vi "FTW-Test-JSON-Fuzz.vi"() -> (0 "Test Result":errorcluster)   [LabVIEW 2015]
uses:
  src/error/FTW-ERR-ThrowInfo.vi
  src/error/FTW-ERR-ThrowError.vi
  src/error/FTW-ERR-CallChain.vi
  src/string/FTW-STR-ReplaceWhitespace.vi
  src/string/FTW-STR-Array-Delimit.vi
  src/error/FTW-ERR-Clear.vi
  src/regex/FTW-Regex-ReplaceAll.vi
  codegen/xnode/FTW-Dataflow-Synchronizer.xnode
panel:
  out "JSON String (UTF-8)":string
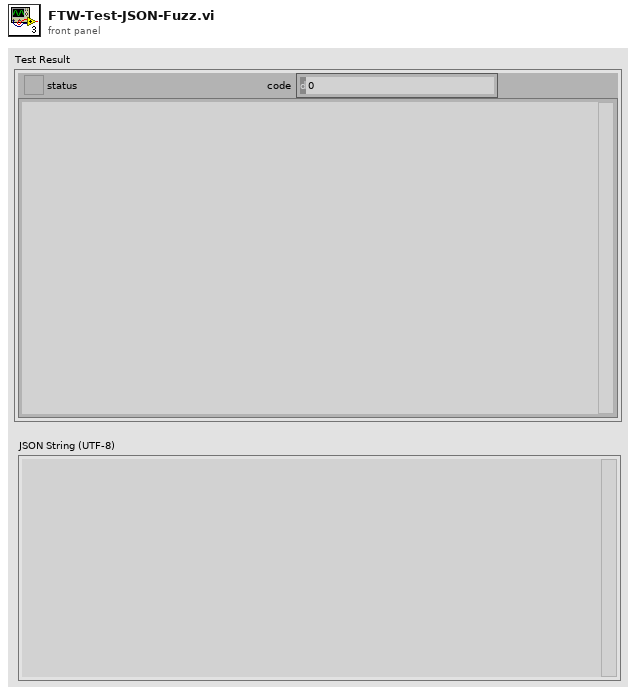
[diagram p1: front panel]
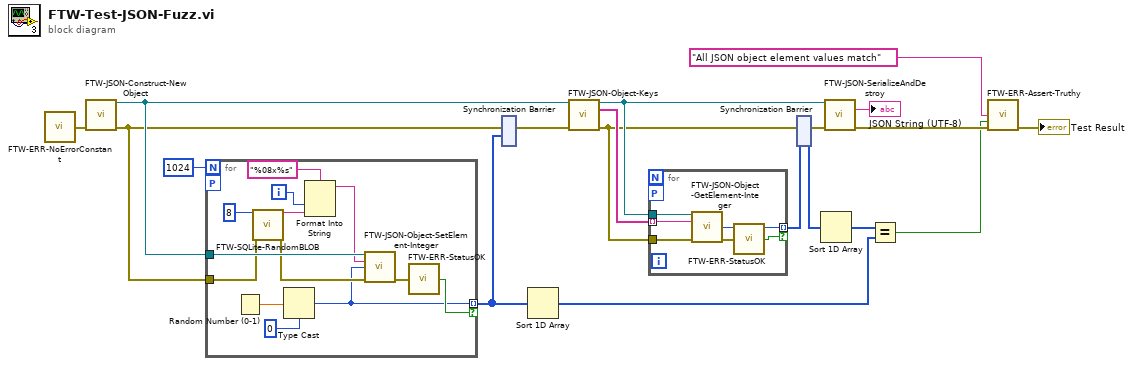
[diagram p0: block diagram]
diagram:
  n1 = call "FTW-ERR-NoErrorConstant.vi"() -> ("no error"=w16:errorcluster)
  n2 = call "FTW-JSON-Construct-NewObject.vi"("error in"=w16) -> ("JSON Object"=w18:refnum<data-value>, "error out"=w9:errorcluster)  [unwired: 13 in]
  n3 = for {
    N: 1024 -> [_]
    workers-P: _ -> [_]
    tunnel: w9 -> [w30]
    tunnel: w18 -> [w32]
    tunnel: [w21] -> w7 mode=indexing if=w23
    i -> [w26]
    n4 = Random Number (0-1)() -> (number: 0 to 1=w22:dbl)
    n5 = call "FTW-SQLite-RandomBLOB.vi"("Number of Bytes"=8, "error in"=w30) -> ("Random BLOB"=w27:string, "error out"=w29:errorcluster)  [unwired: 12 in]
    n6 = Type Cast(type=i64 0, x=w22) -> (*(type *) &x=w21:i64)
    n7 = Format Into String(format string="%08x%s", w26, w27) -> (resulting string=w24:string)  [unwired: 2 in, 1 out]
    n8 = call "FTW-JSON-Object-SetElement-Integer.vi"("JSON Object"=w32, "Key"=w24, "Value"=w21, "error in"=w29) -> ("error out"=w28:errorcluster)  [unwired: 10 in, 1 out]
    n9 = call "FTW-ERR-StatusOK.vi"("error to check"=w28) -> ("Status OK?"=w23:bool)
  }
  n10 = xnode "Synchronization Barrier"("Synchronized Signal 1"=w9, "Synchronized Signal 2"=w7) -> ("error out out"=w8:errorcluster)  [unwired: 1 out]
  n11 = Sort 1D Array(array=w7) -> (sorted array=w13:i64[])
  n12 = call "FTW-JSON-Object-Keys.vi"("JSON Object"=w18, "error in"=w8) -> ("JSON Object out"=w11:refnum<data-value>, "Keys"=w15:string[], "error out"=w6:errorcluster)  [unwired: 11 in]
  n13 = for {
    tunnel: w15 -> [w37] mode=indexing
    tunnel: [w35] -> w4 mode=indexing if=w33
    workers-P: _ -> [_]
    tunnel: w11 -> [w38]
    tunnel: w6 -> [w36]
    n14 = call "FTW-JSON-Object-GetElement-Integer.vi"("JSON Object"=w38, "Key"=w37, "error in"=w36) -> ("Value"=w35:i64, "error out"=w34:errorcluster)  [unwired: 9 in, 2 out]
    n15 = call "FTW-ERR-StatusOK.vi"("error to check"=w34) -> ("Status OK?"=w33:bool)
  }
  n16 = xnode "Synchronization Barrier"("Synchronized Signal 1"=w6, "Synchronized Signal 2"=w4) -> ("error out out"=w5:errorcluster, "out"=w3:i64[])
  n17 = Sort 1D Array(array=w3) -> (sorted array=w14:i64[])
  n18 = call "FTW-JSON-SerializeAndDestroy.vi"("JSON Object"=w11, "error in"=w5) -> ("JSON String (UTF-8)"=→"JSON String (UTF-8)":string, "error out"=w10:errorcluster)  [unwired: 12 in]
  n19 = Equal?(x=w14, y=w13) -> (x = y?=w2:bool)
  n20 = call "FTW-ERR-Assert-Truthy.vi"("Assertion"="All JSON object element values match", "Assertion holds true?"=w2, "error in"=w10) -> ("error out"=→"Test Result":errorcluster)  [unwired: 12 in]
